vi "convTaskStateDateToData.vi"(1 "Variant":variant) -> (0 "data":errorcluster)   [LabVIEW 2010, in "pdbm_task_route.lvlib"]
uses:
  pdbm_task_route.lvlib
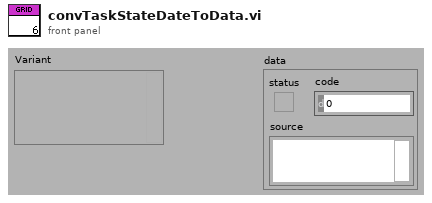
[diagram p1: front panel]
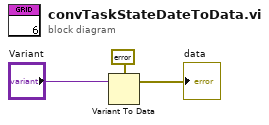
[diagram p0: block diagram]
diagram:
  n1 = Variant To Data(Variant="Variant", type=errorcluster {"status"=FALSE, "code"=0, "source"=""} ("error in (no error)")) -> (data=→"data":errorcluster)  [unwired: 1 in, 1 out]
